vi "FTW-Endpoint-Construct-ZMQ.vi"(5 "Socket Pointer":u64 format="%016x", 11 "error in":errorcluster) -> (4 "FTW ØMQ Endpoint":refnum<class "FTW-Endpoint-ZMQ.lvclass">, 15 "error out":errorcluster)   [LabVIEW 2012, in "FTW-Actor.lvlib" / "FTW-Endpoint-ZMQ.lvclass"]
uses:
  FTW-Endpoint-ZMQ.lvclass
  FTW-Endpoint-ZMQ.lvclass/FTW-Endpoint-ZMQ.ctl
panel:
  # "Inputs"
  # "Outputs"
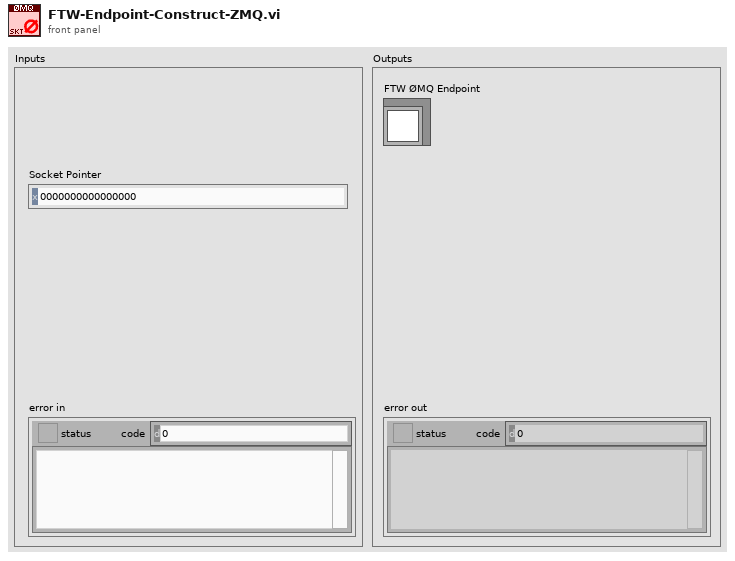
[diagram p1: front panel]
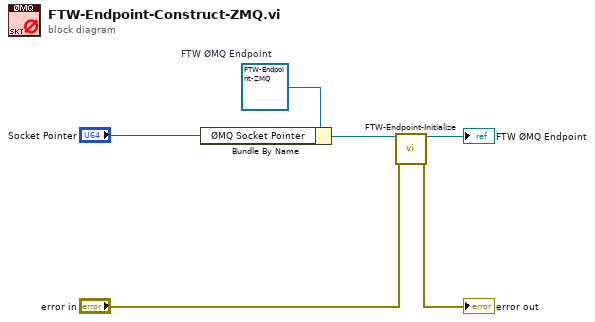
[diagram p0: block diagram]
diagram:
  w6 = refnum<class "FTW-Endpoint-ZMQ.lvclass"> refnum  # FTW ØMQ Endpoint
  n1 = Bundle By Name(cluster=w6, "ØMQ Socket Pointer"="Socket Pointer") -> (w4:refnum<class "FTW-Endpoint-ZMQ.lvclass">)
  n2 = call-dynamic "FTW-Endpoint-Initialize.vi"("FTW Endpoint Type"=w4, "error in"="error in") -> ("FTW Endpoint"=→"FTW ØMQ Endpoint":refnum<class "FTW-Endpoint-ZMQ.lvclass">, "error out"=→"error out":errorcluster)  [unwired: 12 in]
